vi "Format_Regular_Exp.vi"(1 "Regular expression":string) -> (0 "Case Insensitive for html":string)   [LabVIEW 2010]
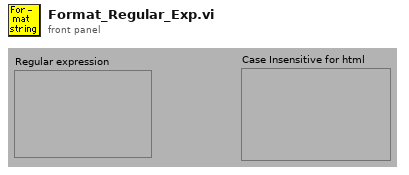
[diagram p1: front panel]
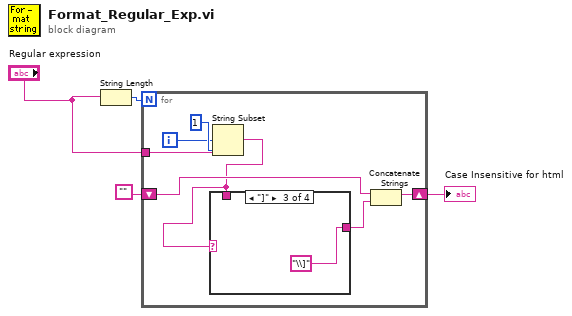
[diagram p0: block diagram]
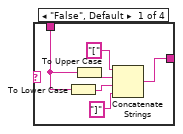
[diagram p2: hidden frame]
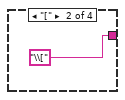
[diagram p3: hidden frame]
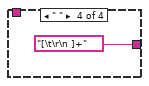
[diagram p4: hidden frame]
diagram:
  n1 = String Length(string="Regular expression") -> (length=w2:i32)
  n2 = for {
    N: w2 -> [_]
    tunnel: "Regular expression" -> [w9]
    shift-right: [w7] -> w1
    shift-left: "" -> [w8]
    i -> [w10]
    n3 = String Subset(string=w9, offset (0)=w10, length (rest)=1 ("length")) -> (substring=w5:string)
    n4 = case shown="\"]\"" w5 {
      tunnel: w5 -> [w17 _ _ _]
      tunnel: [w14 "\\[" "\\]" "[\t\r\n ]+"] -> w6
      frame "False", Default {
        n5 = To Lower Case(string=w17) -> (all lower case string=w15:string)
        n6 = To Upper Case(1:w17) -> (0:w16:string)
        n7 = Concatenate Strings("[", w16, w15, "]" ("Substring")) -> (w14:string)
      }
      frame "[" {
      }
      frame "]" {
      }
      frame " " {
      }
    }
    n8 = Concatenate Strings(w8, w6) -> (w7:string)
  }
  "Case Insensitive for html" <- w1
